vi "WaveformDataStore.vi"(2 "Digitizer Settings":T1, 3 "error in":errorcluster, 4 "Digitizer Data":waveform(dbl)[][](array[waveform]), 5 "Tree DVR In":refnum<data-value>) -> (0 "error out":errorcluster)   [LabVIEW 2014]
uses:
  <vilib>/MDSplus/Classes/Tree_Class/Tree.lvclass
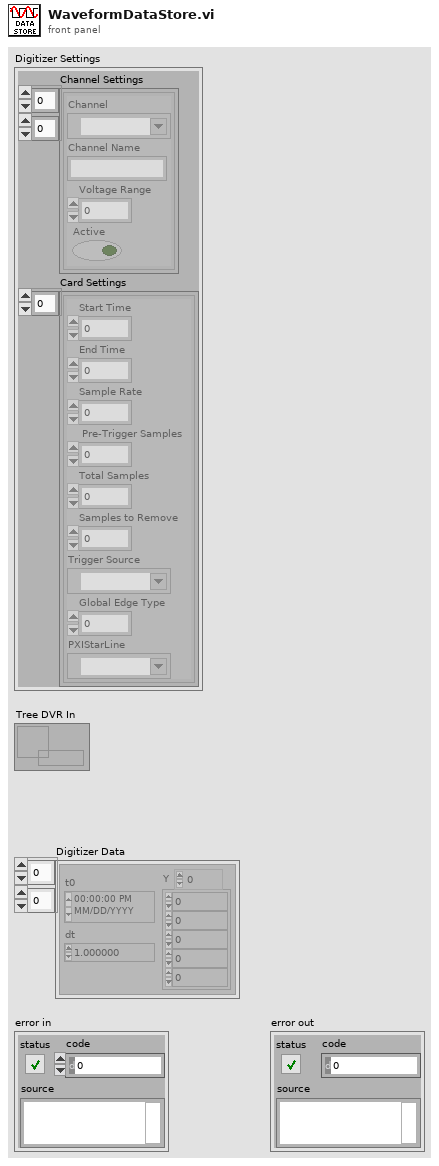
[diagram p1: front panel]
types:
  T1 = cluster{"Channel Settings":cluster{"Channel":tag, "Channel Name":string, "Voltage Range":dbl, "Active":bool}[][], "Card Settings":cluster{"Start Time":dbl, "End Time":dbl, "Sample Rate":dbl, " Pre-Trigger Samples":u32, "Total Samples":i32, "Samples to Remove":u32, "Trigger Source":tag, "Global Edge Type":i32, "PXIStarLine":tag}[]}
  T2 = cluster{"Channel":tag, "Channel Name":string, "Voltage Range":dbl, "Active":bool}[][]
  T3 = cluster{"Start Time":dbl, "End Time":dbl, "Sample Rate":dbl, " Pre-Trigger Samples":u32, "Total Samples":i32, "Samples to Remove":u32, "Trigger Source":tag, "Global Edge Type":i32, "PXIStarLine":tag}[]
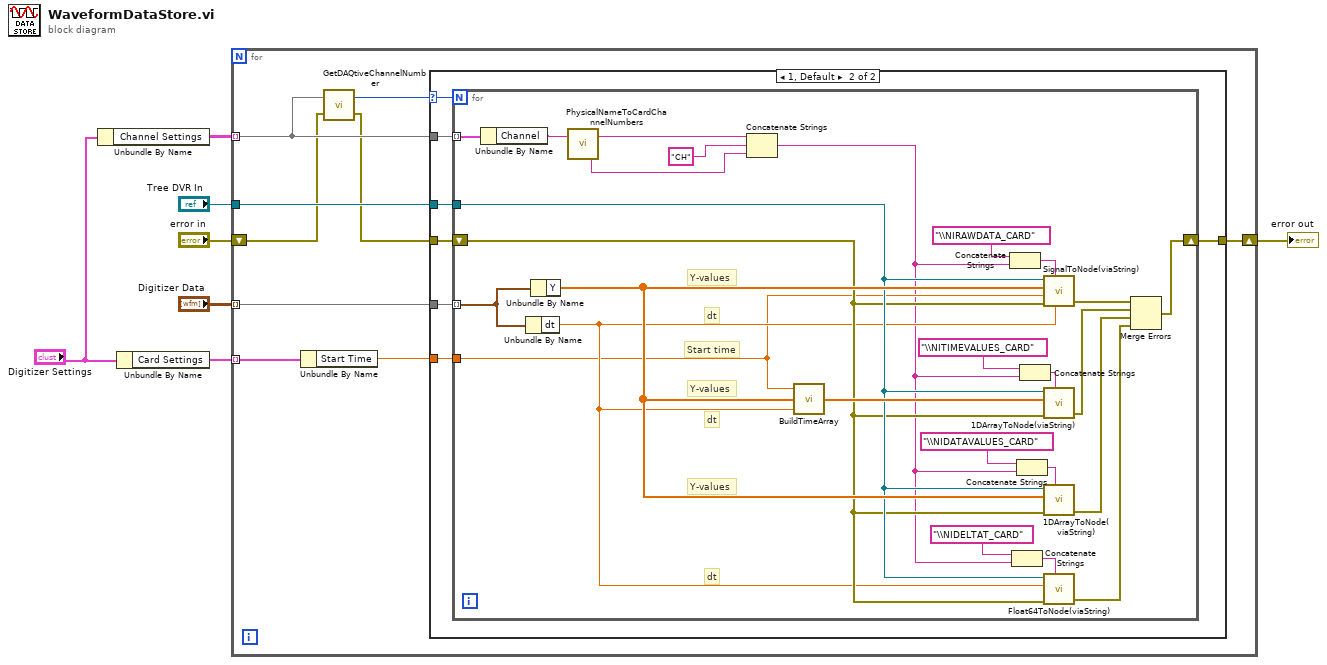
[diagram p0: block diagram]
diagram:
  n1 = Unbundle By Name("Digitizer Settings") -> ("Channel Settings"=w1:T2)
  n2 = Unbundle By Name("Digitizer Settings") -> ("Card Settings"=w2:T3)
  n3 = for {
    tunnel: "Tree DVR In" -> [w12]
    shift-right: [w13] -> w6
    shift-left: "error in" -> [w10]
    tunnel: "Digitizer Data" -> [w14] mode=indexing
    tunnel: w2 -> [w16] mode=indexing
    tunnel: w1 -> [w11] mode=indexing
    n4 = Unbundle By Name(w16) -> ("Start Time"=w15:dbl)
    n5 = call "GetDAQtiveChannelNumber.vi"("error in (no error)"=w10, "Channel Settings"=w11) -> ("error out"=w9:errorcluster, "Numeric"=w8:i32)
    n6 = case shown="1, Default" w8 {
      selector: w8 -> [_ w18]
      tunnel: w15 -> [_ w24]
      tunnel: w14 -> [_ w23]
      tunnel: [w17 w22] -> w13
      tunnel: w12 -> [_ w21]
      tunnel: w11 -> [_ w20]
      tunnel: w9 -> [w17 w19]
      frame 0 {
      }
      frame 1, Default {
        n7 = for {
          N: w18 -> [_]
          tunnel: w23 -> [w50] mode=indexing
          tunnel: w21 -> [w38]
          shift-right: [w47] -> w22
          shift-left: w19 -> [w37]
          tunnel: w24 -> [w34]
          tunnel: w20 -> [w33] mode=indexing
          # "dt"
          # "dt"
          # "Y-values"
          # "Y-values"
          # "Y-values"
          # "dt"
          # "Start time"
          n8 = Unbundle By Name(w33) -> ("Channel"=w32:tag)
          n9 = Unbundle By Name(w50) -> ("dt"=w36:dbl)
          n10 = Unbundle By Name(w50) -> ("Y"=w41:dbl[])
          n11 = call "PhysicalNameToCardChannelNumbers.vi"("NI Physical Channel"=w32) -> ("Channel #"=w30:string, "Card #"=w31:string)  [unwired: 1 in]
          n12 = Concatenate Strings(w31, "CH" ("string"), w30) -> (w25:string)
          n13 = call "BuildTimeArray.vi"("Time Increment (dt)"=w36, "Data Array (y-values)"=w41, "Start Time (t_o)"=w34) -> ("Time Array (x-values)"=w44:dbl[])
          n14 = Concatenate Strings("\\NIRAWDATA_CARD" ("string"), w25) -> (w46:string)
          n15 = Concatenate Strings("\\NIDELTAT_CARD" ("string"), w25) -> (w39:string)
          n16 = Concatenate Strings("\\NIDATAVALUES_CARD" ("string"), w25) -> (w42:string)
          n17 = Concatenate Strings("\\NITIMEVALUES_CARD" ("string"), w25) -> (w45:string)
          n18 = call "SignalToNode(viaString).vi"("Tree DVR in"=w38, "NodePath"=w46, "y-axis (Data Range)"=w41, "Start Time"=w34, "Delta t"=w36, "error in (no error)"=w37) -> ("Error Message Output"=w48:errorcluster)  [unwired: 2 out]
          n19 = call "1DArrayToNode(viaString).vi"("Tree DVR in"=w38, "DBL Array"=w44, "error in (no error)"=w37, "NodePath"=w45) -> ("error out"=w43:errorcluster)  [unwired: 1 in, 2 out]
          n20 = call "1DArrayToNode(viaString).vi"("Tree DVR in"=w38, "DBL Array"=w41, "error in (no error)"=w37, "NodePath"=w42) -> ("error out"=w40:errorcluster)  [unwired: 1 in, 2 out]
          n21 = call "Float64ToNode(viaString).vi"("Tree DVR in"=w38, "DBL in"=w36, "error in"=w37, "NodePath"=w39) -> ("error out"=w35:errorcluster)  [unwired: 1 in, 2 out]
          n22 = Merge Errors(w48, w43, w40, w35) -> (w47:errorcluster)
        }
      }
    }
  }
  "error out" <- w6
